vi "Mitsubishi_Response Message Format.vi"(8 "error in":errorcluster, 11 "Respond Data":string) -> (0 "error out":errorcluster, 3 "Response Message":T1 {"Subheader" format="%.0x"; "Access Route"."Network No." format="%.0x"; "Access Route"."PC No." format="%.0x"; "Access Route"."Module I/O No." format="%.0x"; "Access Route"."Module Station No." format="%.0x"; "End Code" format="%.0x"; "Response Data" format="%.0x"})   [LabVIEW 2018]
uses:
  Data Def/Mitsubishi_Read Response Message.ctl
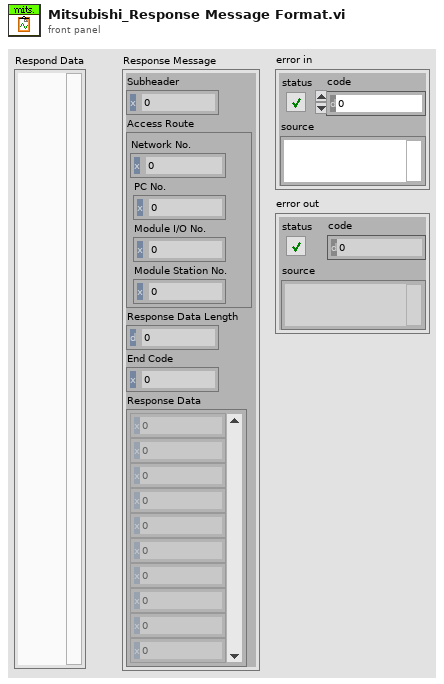
[diagram p1: front panel]
types:
  T1 = typedef "Mitsubishi_Read Response Message.ctl" = cluster{"Subheader":u16, "Access Route":cluster{"Network No.":u8, "PC No.":u8, "Module I/O No.":u16, "Module Station No.":u8}, "Response Data Length":u8, "End Code":u16, "Response Data":i16[]}
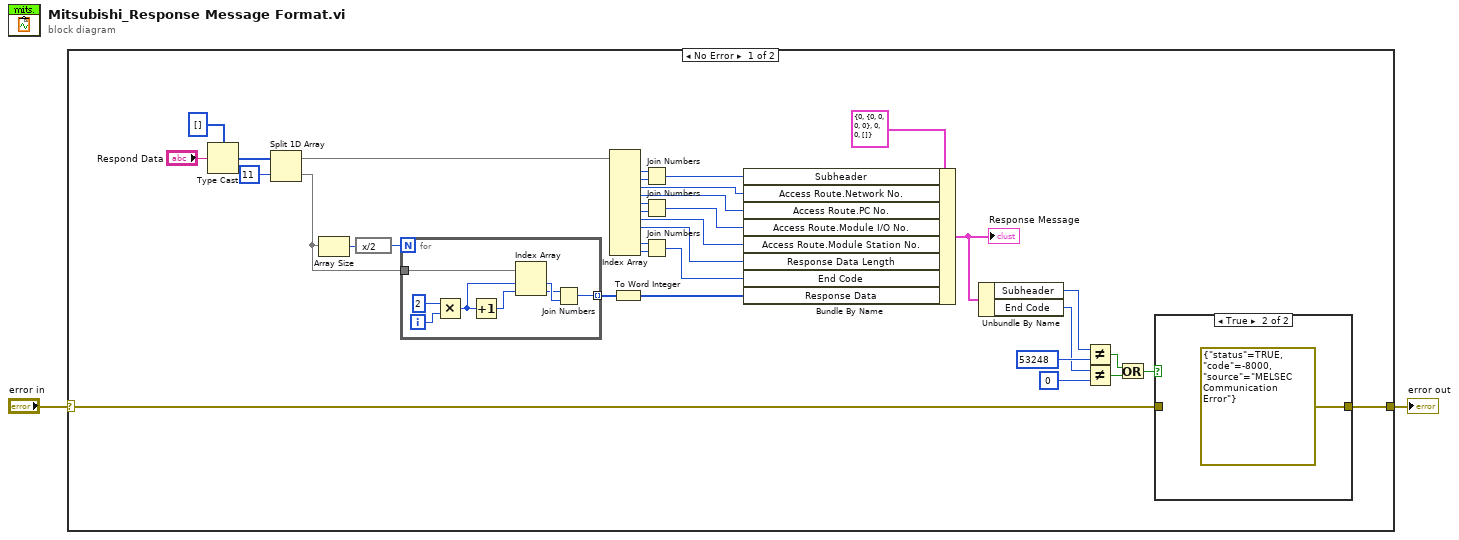
[diagram p0: block diagram]
diagram:
  n1 = case shown="No Error" "error in" {
    selector: "error in" -> [w11 w47]
    tunnel: [w10 w47] -> w1
    frame No Error {
      n2 = Type Cast(type=u8[] [], x="Respond Data") -> (*(type *) &x=w22:u8[])
      n3 = Split 1D Array(array=w22, index=11) -> (first subarray=w20:u8[], second subarray=w7:u8[])
      n4 = Array Size(array=w7) -> (size(s)=w6:i32)
      n5 = expression code="x/2"(w6) -> (w5:i32)
      n6 = for {
        N: w5 -> [_]
        tunnel: w7 -> [w44]
        tunnel: [w37] -> w4 mode=indexing
        i -> [w43]
        n7 = Multiply(x=2, y=w43) -> (x*y=w41:i32)
        n8 = Increment(x=w41) -> (x+1=w40:i32)
        n9 = Index Array(array=w44, index #1=w41, index #2=w40) -> (element #1=w39:u8, element #2=w38:u8)
        n10 = Join Numbers(hi=w38, lo=w39) -> ((hi.lo)=w37:u16)
      }
      n11 = Index Array(array=w20) -> (element #1=w34:u8, element #2=w33:u8, element #3=w31:u8, element #4=w30:u8, element #5=w29:u8, element #6=w28:u8, element #7=w26:u8, element #8=w19:u8, element #10=w24:u8, element #11=w25:u8)  [unwired: 11 in, 1 out]
      n12 = To Word Integer(number=w4) -> (16bit integer=w3:i16[])
      n13 = Join Numbers(hi=w34, lo=w33) -> ((hi.lo)=w32:u16)
      n14 = Join Numbers(hi=w29, lo=w28) -> ((hi.lo)=w27:u16)
      n15 = Join Numbers(hi=w24, lo=w25) -> ((hi.lo)=w23:u16)
      n16 = Bundle By Name(cluster=T1 {"Subheader"=0, "Access Route"={"Network No."=0, "PC No."=0, "Module I/O No."=0, "Module Station No."=0}, "Response Data Length"=0, "End Code"=0, "Response Data"=[]} ("Response Message"), "Subheader"=w32, "Access Route.Network No."=w31, "Access Route.PC No."=w30, "Access Route.Module I/O No."=w27, "Access Route.Module Station No."=w26, "Response Data Length"=w19, "End Code"=w23, "Response Data"=w3) -> (w8:T1)
      "Response Message" <- w8
      n17 = Unbundle By Name(w8) -> ("Subheader"=w18:u16, "End Code"=w16:u16)
      n18 = Not Equal?(x=w18, y=u16 53248) -> (x != y?=w13:bool)
      n19 = Not Equal?(x=w16, y=u16 0) -> (x != y?=w14:bool)
      n20 = Or(x=w13, y=w14) -> (x .or. y?=w12:bool)
      n21 = case shown="True" w12 {
        tunnel: w11 -> [w45 _]
        tunnel: [w45 errorcluster {"status"=TRUE, "code"=-8000, "source"="MELSEC Communication Error"} ("error IO")] -> w10
        frame False {
        }
        frame True {
        }
      }
    }
    frame Error {
    }
  }
  "error out" <- w1
